vi "Phi.vi"(6 "Number":i32, 7 "STD":dbl, 9 "x_f":dbl, 10 "x_0":dbl, 11 "Output (mm)":dbl) -> (3 "Array":dbl[](array[numeric]))   [LabVIEW 2021]
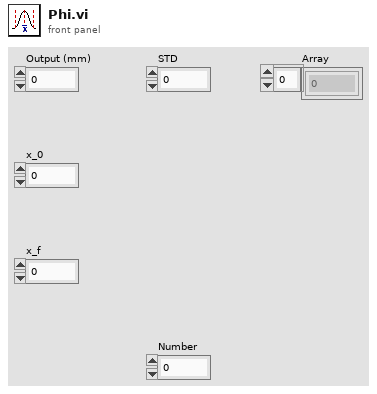
[diagram p1: front panel]
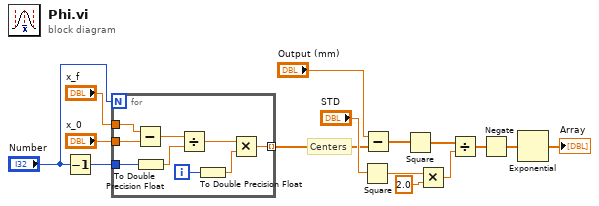
[diagram p0: block diagram]
diagram:
  # "Centers"
  n1 = Decrement(x="Number") -> (x-1=w4:i32)
  n2 = for {
    N: "Number" -> [_]
    tunnel: "x_f" -> [w24]
    tunnel: "x_0" -> [w22]
    tunnel: [w23] -> w12 mode=indexing
    tunnel: w4 -> [w16]
    i -> [w18]
    n3 = Subtract(x=w24, y=w22) -> (x-y=w21:dbl)
    n4 = To Double Precision Float(number=w16) -> (double precision float=w19:dbl)
    n5 = Divide(x=w21, y=w19) -> (x/y=w20:dbl)
    n6 = To Double Precision Float(number=w18) -> (double precision float=w17:dbl)
    n7 = Multiply(x=w20, y=w17) -> (x*y=w23:dbl)
  }
  n8 = Square(x="STD") -> (x^2=w1:dbl)
  n9 = Subtract(x="Output (mm)", y=w12) -> (x-y=w5:dbl[])
  n10 = Square(x=w5) -> (x^2=w6:dbl[])
  n11 = Multiply(x=w1, y=2.0) -> (x*y=w15:dbl)
  n12 = Divide(x=w6, y=w15) -> (x/y=w7:dbl[])
  n13 = Negate(x=w7) -> (-x=w8:dbl[])
  n14 = Exponential(1:w8) -> (0:→"Array":dbl[])
